vi "full.vi"() -> ()   [LabVIEW 2017]
uses:
  <vilib>/myRIO/Instrument Drivers/Onboard IO/DIO/typedefs/DIO Reference.ctl
  <vilib>/myRIO/Common/Instrument Driver Framework/Utilities/typedefs/myRIO Generic Hardware Reference.ctl
  <vilib>/myRIO/Common/Instrument Driver Framework/Utilities/typedefs/Hardware Version Enum.ctl
  <vilib>/myRIO/Common/Instrument Driver Framework/Utilities/typedefs/myRIO v1.0 Reference.ctl
  <vilib>/myRIO/Common/Instrument Driver Framework/Utilities/typedefs/Generic FPGA Reference.ctl
  <vilib>/myRIO/Common/Instrument Driver Framework/myRIO v1.0/DIO/typedefs/DIO Channels List.ctl
  <vilib>/myRIO/Common/Instrument Driver Framework/myRIO v1.0/DIO/typedefs/DIO Channels Enum.ctl
  <vilib>/userdefined/High Color/nirio_resource_hc.ctl
  <vilib>/myRIO/Common/Instrument Driver Framework/Utilities/vis/Is FPGA Ref Available.vi
  <vilib>/myRIO/Common/Instrument Driver Framework/myRIO v1.0/DIO/vis/myRIO v1.1 Open DIO.vi
  <vilib>/myRIO/Instrument Drivers/Onboard IO/DIO/vis/Write.vi
  <vilib>/myRIO/Common/Instrument Driver Framework/Utilities/vis/Validate Channels.vi
  <vilib>/myRIO/Common/Instrument Driver Framework/myRIO v1.0/DIO/vis/myRIO v1.0 Reserve DIO.vi
  <vilib>/myRIO/Common/Instrument Driver Framework/myRIO v1.0/UART/vis/myRIO v1.0 Close UART.vi
  <vilib>/myRIO/Common/Instrument Driver Framework/myRIO v1.0/Resource Manager/vis/myRIO v1.0 Reserve Channel List.vi
  <vilib>/myRIO/Common/Instrument Driver Framework/myRIO v1.0/DIO/vis/myRIO v1.0 Build MUX Configuration DIO.vi
  <vilib>/myRIO/Common/Instrument Driver Framework/myRIO v1.0/Resource Manager/vis/myRIO v1.0 Reserve Channel.vi
  <vilib>/myRIO/Common/Instrument Driver Framework/myRIO v1.0/Resource Manager/vis/myRIO v1.0 Unreserve Channel.vi
  <vilib>/myRIO/Common/Instrument Driver Framework/myRIO v1.0/Resource Manager/vis/myRIO v1.0 Create Configuration List.vi
  <vilib>/myRIO/Common/Instrument Driver Framework/myRIO v1.0/Resource Manager/vis/myRIO v1.0 Build Mutex Name.vi
  <vilib>/Utility/VariantDataType/GetNumericInfo.vi
  <vilib>/Utility/error.llb/Error Cluster From Error Code.vi
  <vilib>/myRIO/Common/Instrument Driver Framework/myRIO v1.0/myRIO v1.1 Open.vi
  <vilib>/myRIO/Common/Instrument Driver Framework/Utilities/vis/IO Manager.vi
  <vilib>/myRIO/Common/Instrument Driver Framework/Utilities/vis/Configuration Manager.vi
  <vilib>/myRIO/Common/Instrument Driver Framework/myRIO v1.0/Resource Manager/vis/myRIO v1.0 Configure IO.vi
  <vilib>/myRIO/Common/Instrument Driver Framework/myRIO v1.0/myRIO v1.0 Close.vi
  <vilib>/myRIO/Common/Instrument Driver Framework/myRIO v1.0/DIO/vis/myRIO v1.0 Write DIO.vi
  <vilib>/myRIO/Common/Instrument Driver Framework/Utilities/vis/FPGA Ref Manager.vi
  <vilib>/myRIO/Common/Instrument Driver Framework/myRIO v1.0/myRIO v1.0 Reset FPGA.vi
  <vilib>/myRIO/Common/Instrument Driver Framework/myRIO v1.0/IRQ/vis/myRIO v1.0 IRQ Info FGV.vi
  <vilib>/myRIO/Common/Instrument Driver Framework/myRIO v1.0/IRQ/vis/myRIO v1.0 Timer IRQ Info FGV.vi
  <vilib>/myRIO/Common/Instrument Driver Framework/myRIO v1.0/IRQ/vis/myRIO v1.0 ISR Agent.vi
  <vilib>/myRIO/Express VI/Onboard Devices/LED/LED Express VI.xnode
  <vilib>/myRIO/Instrument Drivers/Onboard IO/DIO/vis/myRIO DIO Open.xnode
  <vilib>/myRIO/Instrument Drivers/Utilities/Utilities.lvlib
  <vilib>/myRIO/Instrument Drivers/Onboard IO/DIO/DIO.lvlib
panel:
  in  "state":T1(ring)
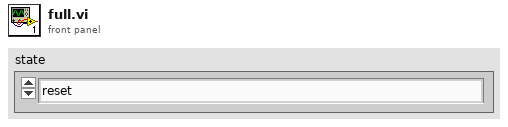
[diagram p1: front panel]
types:
  T1 = enum16{"reset", "M2 -> tunnel -> M5", "M1 -> tunnel -> M3", "rotate 360 angle", "meter back", "meter forward", "tunnel -> M5 crossing pool", "tunnel -> M5"}
  T2 = typedef "DIO.lvlib/DIO Reference.ctl" = cluster{"myRIO Reference":T3, "DIO Channels List":T7}
  T3 = typedef "myRIO Generic Hardware Reference.ctl" = cluster{"myRIO Model":T4, "myRIO Hardware Reference":T5}
  T4 = typedef "Hardware Version Enum.ctl" = enum16{"Unknown", "myRIO-1900", "myRIO-1950", "roboRIO", "NI ELVIS RIO CM"}
  T5 = typedef "myRIO v1.0 Reference.ctl" = cluster{"Generic FPGA Reference":T6, "Allow multiple opens":bool}
  T6 = typedef "Generic FPGA Reference.ctl" = refnum<k20>
  T7 = typedef "DIO Channels List.ctl" = T8[]
  T8 = typedef "DIO Channels Enum.ctl" = enum16{"Not Connected", "C/DIO0", "C/DIO1", "C/DIO2", "C/DIO3", "C/DIO4", "C/DIO5", "C/DIO6", "C/DIO7", "A/DIO0", "A/DIO1", "A/DIO2", "A/DIO3", "A/DIO4", "A/DIO5", "A/DIO6", "A/DIO7", "A/DIO8", "A/DIO9", "A/DIO10", "A/DIO11", "A/DIO12", "A/DIO13", "A/DIO14", "A/DIO15", "B/DIO0", "B/DIO1", "B/DIO2", "B/DIO3", "B/DIO4", "B/DIO5", "B/DIO6", "B/DIO7", "B/DIO8", "B/DIO9", "B/DIO10", "B/DIO11", "B/DIO12", "B/DIO13", "B/DIO14", "B/DIO15", "LED0", "LED1", "LED2", "LED3", "Button0", "DIO/DIO0", "DIO/DIO1", "DIO/DIO2", "DIO/DIO3", "DIO/DIO4", "DIO/DIO5", "DIO/DIO6", "DIO/DIO7", "DIO/DIO8", "DIO/DIO9", "SPI/CS0", "SPI/CS1", "SPI/CS2", "SPI/CS3", "LED RADIO (Green)", "LED RADIO (Red)", "LED COMM (Green)", "LED COMM (Red)", "LED MODE (Green)", "LED MODE (Red)"}
  T9 = typedef "nirio_resource_hc.ctl" = tag
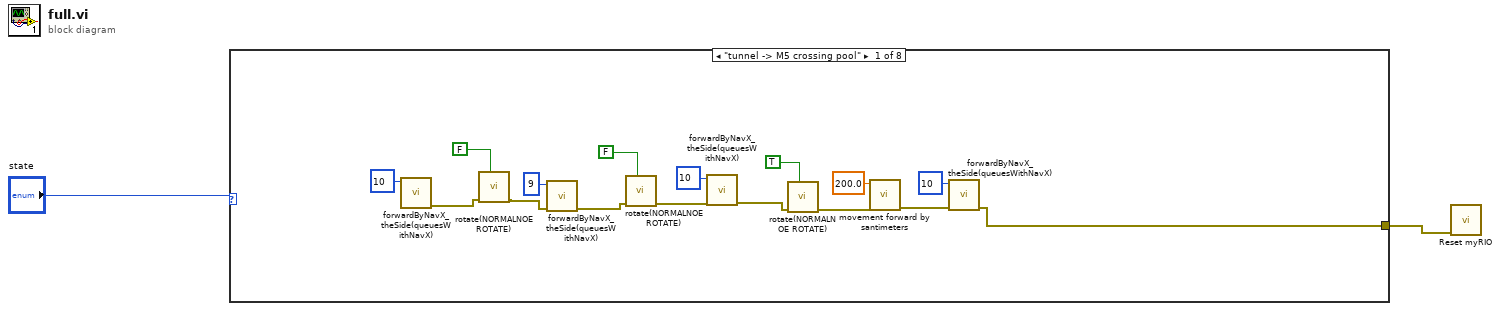
[diagram p0: block diagram]
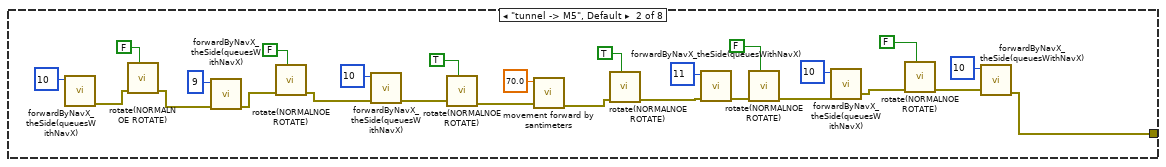
[diagram p2: hidden frame]
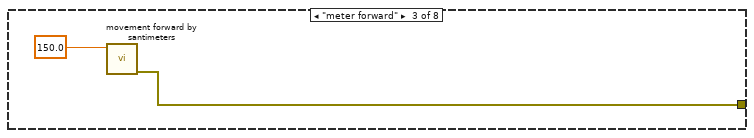
[diagram p3: hidden frame]
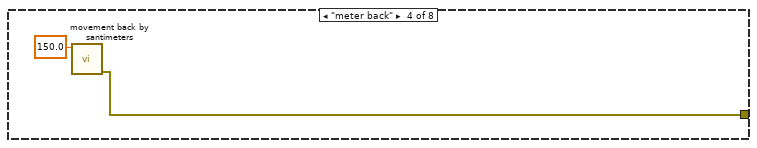
[diagram p4: hidden frame]
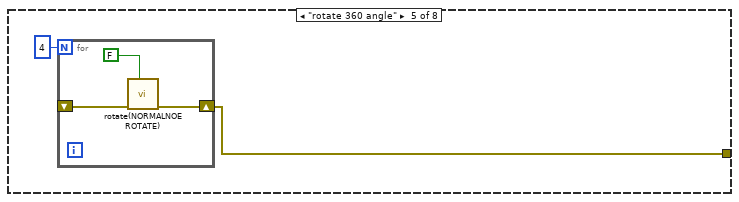
[diagram p5: hidden frame]
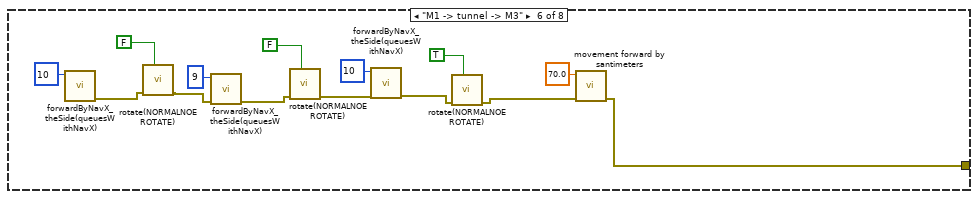
[diagram p6: hidden frame]
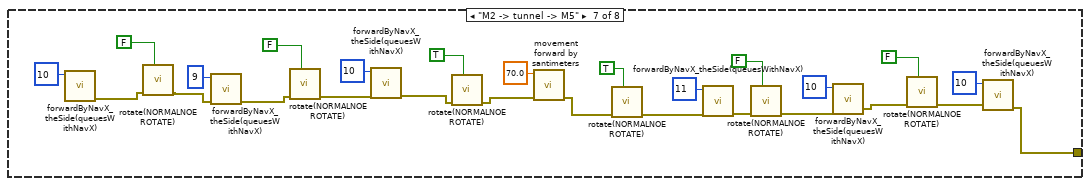
[diagram p7: hidden frame]
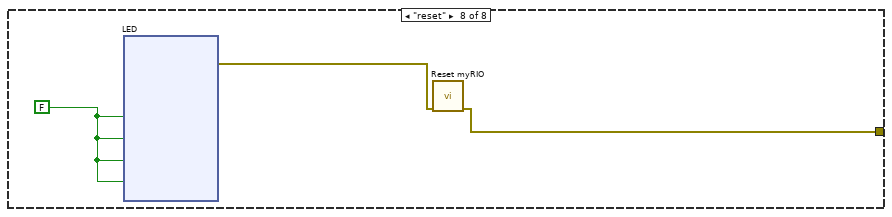
[diagram p8: hidden frame]
diagram:
  n1 = case shown="\"tunnel -> M5 crossing pool\"" "state" {
    tunnel: [w3 w19 w45 w48 w49 w54 w68 w96] -> w1
    frame "tunnel -> M5 crossing pool" {
      n2 = call "forwardByNavX_theSide(queuesWithNavX).vi"("distance the side"=u32 10) -> ("error out"=w15:errorcluster)  [unwired: 9 in, 1 out]
      n3 = call "rotate(NORMALNOE ROTATE).vi"("On/Off\nRight/Left"=FALSE ("On/Off\nRight/Left"), "error in (no error)"=w15) -> ("error out"=w14:errorcluster)  [unwired: 8 in, 1 out]
      n4 = call "forwardByNavX_theSide(queuesWithNavX).vi"("error in (no error)"=w14, "distance the side"=u32 9) -> ("error out"=w12:errorcluster)  [unwired: 8 in, 1 out]
      n5 = call "rotate(NORMALNOE ROTATE).vi"("On/Off\nRight/Left"=FALSE ("On/Off\nRight/Left"), "error in (no error)"=w12) -> ("error out"=w13:errorcluster)  [unwired: 8 in, 1 out]
      n6 = call "forwardByNavX_theSide(queuesWithNavX).vi"("error in (no error)"=w13, "distance the side"=u32 10) -> ("error out"=w11:errorcluster)  [unwired: 8 in, 1 out]
      n7 = call "rotate(NORMALNOE ROTATE).vi"("On/Off\nRight/Left"=TRUE ("On/Off\nRight/Left"), "error in (no error)"=w11) -> ("error out"=w4:errorcluster)  [unwired: 8 in, 1 out]
      n8 = call "movement forward by santimeters.vi"("error in (no error)"=w4, "distance (cm)"=200.0 ("range in santimeters")) -> ("error out"=w5:errorcluster)  [unwired: 8 in, 1 out]
      n9 = call "forwardByNavX_theSide(queuesWithNavX).vi"("error in (no error)"=w5, "distance the side"=u32 10) -> ("error out"=w3:errorcluster)  [unwired: 8 in, 1 out]
    }
    frame "tunnel -> M5", Default {
      n10 = call "forwardByNavX_theSide(queuesWithNavX).vi"("distance the side"=u32 10) -> ("error out"=w36:errorcluster)  [unwired: 9 in, 1 out]
      n11 = call "rotate(NORMALNOE ROTATE).vi"("On/Off\nRight/Left"=FALSE ("On/Off\nRight/Left"), "error in (no error)"=w36) -> ("error out"=w35:errorcluster)  [unwired: 8 in, 1 out]
      n12 = call "forwardByNavX_theSide(queuesWithNavX).vi"("error in (no error)"=w35, "distance the side"=u32 9) -> ("error out"=w34:errorcluster)  [unwired: 8 in, 1 out]
      n13 = call "rotate(NORMALNOE ROTATE).vi"("On/Off\nRight/Left"=FALSE ("On/Off\nRight/Left"), "error in (no error)"=w34) -> ("error out"=w33:errorcluster)  [unwired: 8 in, 1 out]
      n14 = call "forwardByNavX_theSide(queuesWithNavX).vi"("error in (no error)"=w33, "distance the side"=u32 10) -> ("error out"=w32:errorcluster)  [unwired: 8 in, 1 out]
      n15 = call "rotate(NORMALNOE ROTATE).vi"("On/Off\nRight/Left"=TRUE ("On/Off\nRight/Left"), "error in (no error)"=w32) -> ("error out"=w31:errorcluster)  [unwired: 8 in, 1 out]
      n16 = call "movement forward by santimeters.vi"("error in (no error)"=w31, "distance (cm)"=70.0 ("range in santimeters")) -> ("error out"=w27:errorcluster)  [unwired: 8 in, 1 out]
      n17 = call "rotate(NORMALNOE ROTATE).vi"("On/Off\nRight/Left"=TRUE ("On/Off\nRight/Left"), "error in (no error)"=w27) -> ("error out"=w26:errorcluster)  [unwired: 8 in, 1 out]
      n18 = call "forwardByNavX_theSide(queuesWithNavX).vi"("error in (no error)"=w26, "distance the side"=u32 11) -> ("error out"=w25:errorcluster)  [unwired: 8 in, 1 out]
      n19 = call "rotate(NORMALNOE ROTATE).vi"("On/Off\nRight/Left"=FALSE ("On/Off\nRight/Left"), "error in (no error)"=w25) -> ("error out"=w24:errorcluster)  [unwired: 8 in, 1 out]
      n20 = call "forwardByNavX_theSide(queuesWithNavX).vi"("error in (no error)"=w24, "distance the side"=u32 10) -> ("error out"=w22:errorcluster)  [unwired: 8 in, 1 out]
      n21 = call "rotate(NORMALNOE ROTATE).vi"("On/Off\nRight/Left"=FALSE ("On/Off\nRight/Left"), "error in (no error)"=w22) -> ("error out"=w21:errorcluster)  [unwired: 8 in, 1 out]
      n22 = call "forwardByNavX_theSide(queuesWithNavX).vi"("error in (no error)"=w21, "distance the side"=u32 10) -> ("error out"=w19:errorcluster)  [unwired: 8 in, 1 out]
    }
    frame "meter forward" {
      n23 = call "movement forward by santimeters.vi"("distance (cm)"=150.0 ("range in santimeters")) -> ("error out"=w45:errorcluster)  [unwired: 9 in, 1 out]
    }
    frame "meter back" {
      n24 = call "movement back by santimeters.vi"("range in santimeters"=150.0) -> ("error out"=w48:errorcluster)  [unwired: 10 in]
    }
    frame "rotate 360 angle" {
      n25 = for {
        N: 4 -> [_]
        shift-right: [w52] -> w49
        shift-left: _ -> [w51]
        n26 = call "rotate(NORMALNOE ROTATE).vi"("On/Off\nRight/Left"=FALSE ("On/Off\nRight/Left"), "error in (no error)"=w51) -> ("error out"=w52:errorcluster)  [unwired: 8 in, 1 out]
      }
    }
    frame "M1 -> tunnel -> M3" {
      n27 = call "forwardByNavX_theSide(queuesWithNavX).vi"("distance the side"=u32 10) -> ("error out"=w64:errorcluster)  [unwired: 9 in, 1 out]
      n28 = call "rotate(NORMALNOE ROTATE).vi"("On/Off\nRight/Left"=FALSE ("On/Off\nRight/Left"), "error in (no error)"=w64) -> ("error out"=w63:errorcluster)  [unwired: 8 in, 1 out]
      n29 = call "forwardByNavX_theSide(queuesWithNavX).vi"("error in (no error)"=w63, "distance the side"=u32 9) -> ("error out"=w61:errorcluster)  [unwired: 8 in, 1 out]
      n30 = call "rotate(NORMALNOE ROTATE).vi"("On/Off\nRight/Left"=FALSE ("On/Off\nRight/Left"), "error in (no error)"=w61) -> ("error out"=w62:errorcluster)  [unwired: 8 in, 1 out]
      n31 = call "forwardByNavX_theSide(queuesWithNavX).vi"("error in (no error)"=w62, "distance the side"=u32 10) -> ("error out"=w60:errorcluster)  [unwired: 8 in, 1 out]
      n32 = call "rotate(NORMALNOE ROTATE).vi"("On/Off\nRight/Left"=TRUE ("On/Off\nRight/Left"), "error in (no error)"=w60) -> ("error out"=w55:errorcluster)  [unwired: 8 in, 1 out]
      n33 = call "movement forward by santimeters.vi"("error in (no error)"=w55, "distance (cm)"=70.0 ("range in santimeters")) -> ("error out"=w54:errorcluster)  [unwired: 8 in, 1 out]
    }
    frame "M2 -> tunnel -> M5" {
      n34 = call "forwardByNavX_theSide(queuesWithNavX).vi"("distance the side"=u32 10) -> ("error out"=w90:errorcluster)  [unwired: 9 in, 1 out]
      n35 = call "rotate(NORMALNOE ROTATE).vi"("On/Off\nRight/Left"=FALSE ("On/Off\nRight/Left"), "error in (no error)"=w90) -> ("error out"=w89:errorcluster)  [unwired: 8 in, 1 out]
      n36 = call "forwardByNavX_theSide(queuesWithNavX).vi"("error in (no error)"=w89, "distance the side"=u32 9) -> ("error out"=w87:errorcluster)  [unwired: 8 in, 1 out]
      n37 = call "rotate(NORMALNOE ROTATE).vi"("On/Off\nRight/Left"=FALSE ("On/Off\nRight/Left"), "error in (no error)"=w87) -> ("error out"=w88:errorcluster)  [unwired: 8 in, 1 out]
      n38 = call "forwardByNavX_theSide(queuesWithNavX).vi"("error in (no error)"=w88, "distance the side"=u32 10) -> ("error out"=w86:errorcluster)  [unwired: 8 in, 1 out]
      n39 = call "rotate(NORMALNOE ROTATE).vi"("On/Off\nRight/Left"=TRUE ("On/Off\nRight/Left"), "error in (no error)"=w86) -> ("error out"=w81:errorcluster)  [unwired: 8 in, 1 out]
      n40 = call "movement forward by santimeters.vi"("error in (no error)"=w81, "distance (cm)"=70.0 ("range in santimeters")) -> ("error out"=w69:errorcluster)  [unwired: 8 in, 1 out]
      n41 = call "rotate(NORMALNOE ROTATE).vi"("On/Off\nRight/Left"=TRUE ("On/Off\nRight/Left"), "error in (no error)"=w69) -> ("error out"=w76:errorcluster)  [unwired: 8 in, 1 out]
      n42 = call "forwardByNavX_theSide(queuesWithNavX).vi"("error in (no error)"=w76, "distance the side"=u32 11) -> ("error out"=w75:errorcluster)  [unwired: 8 in, 1 out]
      n43 = call "rotate(NORMALNOE ROTATE).vi"("On/Off\nRight/Left"=FALSE ("On/Off\nRight/Left"), "error in (no error)"=w75) -> ("error out"=w74:errorcluster)  [unwired: 8 in, 1 out]
      n44 = call "forwardByNavX_theSide(queuesWithNavX).vi"("error in (no error)"=w74, "distance the side"=u32 10) -> ("error out"=w72:errorcluster)  [unwired: 8 in, 1 out]
      n45 = call "rotate(NORMALNOE ROTATE).vi"("On/Off\nRight/Left"=FALSE ("On/Off\nRight/Left"), "error in (no error)"=w72) -> ("error out"=w71:errorcluster)  [unwired: 8 in, 1 out]
      n46 = call "forwardByNavX_theSide(queuesWithNavX).vi"("error in (no error)"=w71, "distance the side"=u32 10) -> ("error out"=w68:errorcluster)  [unwired: 8 in, 1 out]
    }
    frame "reset" {
      w94 = FALSE
      n47 = xnode "LED"("LED0"=w94, "LED1"=w94, "LED2"=w94, "LED3"=w94) -> ("error out"=w95:errorcluster)  [unwired: 1 in]
      n48 = call <vilib>:"Reset myRIO.vi"("error in (no error)"=w95) -> ("error out"=w96:errorcluster)  [unwired: 10 in]
    }
  }
  n49 = call <vilib>:"Reset myRIO.vi"("error in (no error)"=w1) -> ()  [unwired: 10 in, 1 out]
